vi "Obtain Request Events.vi"(8 "error in":errorcluster, 10 "Create New? (F)":bool, 11 "Module ID":i32=-1) -> (0 "error out":errorcluster, 2 "RaspberryPiPico Request Events":T1)   [LabVIEW 2024, in "RaspberryPiPico.lvlib"]
doc: "This VI Obtains/Creates the Requests events that will be used for other modules to communicate with the module that owns this VI. These Requests events will be accessed only via Public API methods for this module.\n\n<b>NOTE</b>: The contents of this VI are automatically generated and modified by the <b>Tools > DQMH Consortium > DQMH</b> utilities. Consider using those utilities instead of making your own modifications to this VI.\n_____\nBased on DQMH Dev Tools: Project Template 7.1.0.1503."
uses:
  RaspberryPiPico.lvlib
  Request Events--cluster.ctl
  Stop Argument--cluster.ctl
  Show Panel Argument--cluster.ctl
  Hide Panel Argument--cluster.ctl
  Show Diagram Argument--cluster.ctl
  Get Module Execution Status Argument--cluster.ctl
  Initialize Instrument Argument--cluster.ctl
  Initialize Instrument (Reply Payload)--cluster.ctl
  <instrlib>/HandsOnPi2040/cti-drivers-lv-visa-main/CTI-Visa/Identity.ctl
  Local Instance Request Events--cluster.ctl
  Start Continuous Acquisition Argument--cluster.ctl
  <instrlib>/HandsOnPi2040/cti-drivers-lv-visa-main/CTI-Visa/CTI-Visa.lvlib
  Local Instance Events SEQ/Local Instance Events SEQ.lvlib
panel:
  # "NOTE: The contents of this VI are automatically generated and modified by the Tools > DQMH Consortium > DQMH utilities. Consider using those utilities instead of making your own modifications to this VI."
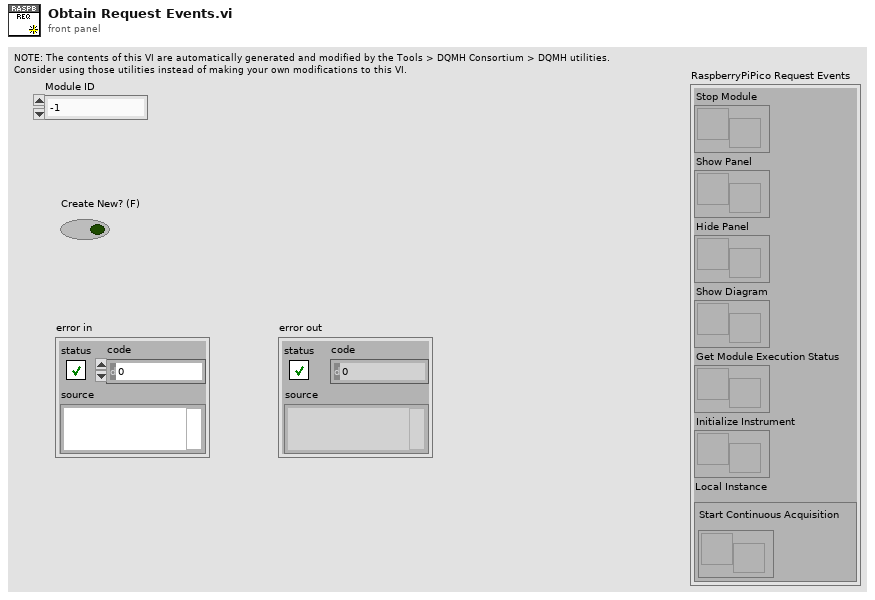
[diagram p1: front panel]
types:
  T1 = typedef "RaspberryPiPico.lvlib/Request Events--cluster.ctl" = cluster{"Stop Module":refnum<user-event>, "Show Panel":refnum<user-event>, "Hide Panel":refnum<user-event>, "Show Diagram":refnum<user-event>, "Get Module Execution Status":refnum<user-event>, "Initialize Instrument":refnum<user-event>, "Local Instance":T2}
  T2 = typedef "RaspberryPiPico.lvlib/Local Instance Request Events--cluster.ctl" = cluster{"Start Continuous Acquisition":refnum<user-event>}
  T3 = typedef "RaspberryPiPico.lvlib/Initialize Instrument Argument--cluster.ctl" = cluster{"Module ID":i32, "VISA resource name":refnum<visa-resource-name>, "Wait Notifier":refnum<notifier>, "wait for reply":bool}
  T4 = typedef "RaspberryPiPico.lvlib/Get Module Execution Status Argument--cluster.ctl" = cluster{"Module ID":i32, "Running?":bool}
  T5 = typedef "RaspberryPiPico.lvlib/Show Diagram Argument--cluster.ctl" = cluster{"Module ID":i32, "Debug?":bool}
  T6 = typedef "RaspberryPiPico.lvlib/Show Panel Argument--cluster.ctl" = cluster{"Module ID":i32, "Show Panel?":bool}
  T7 = typedef "RaspberryPiPico.lvlib/Hide Panel Argument--cluster.ctl" = cluster{"Module ID":i32, "Hide Panel?":bool}
  T8 = typedef "RaspberryPiPico.lvlib/Stop Argument--cluster.ctl" = cluster{"Module ID":i32, "Origin":string, "Exit via Stop Module Req?":bool, "Wait for Module to stop?":bool}
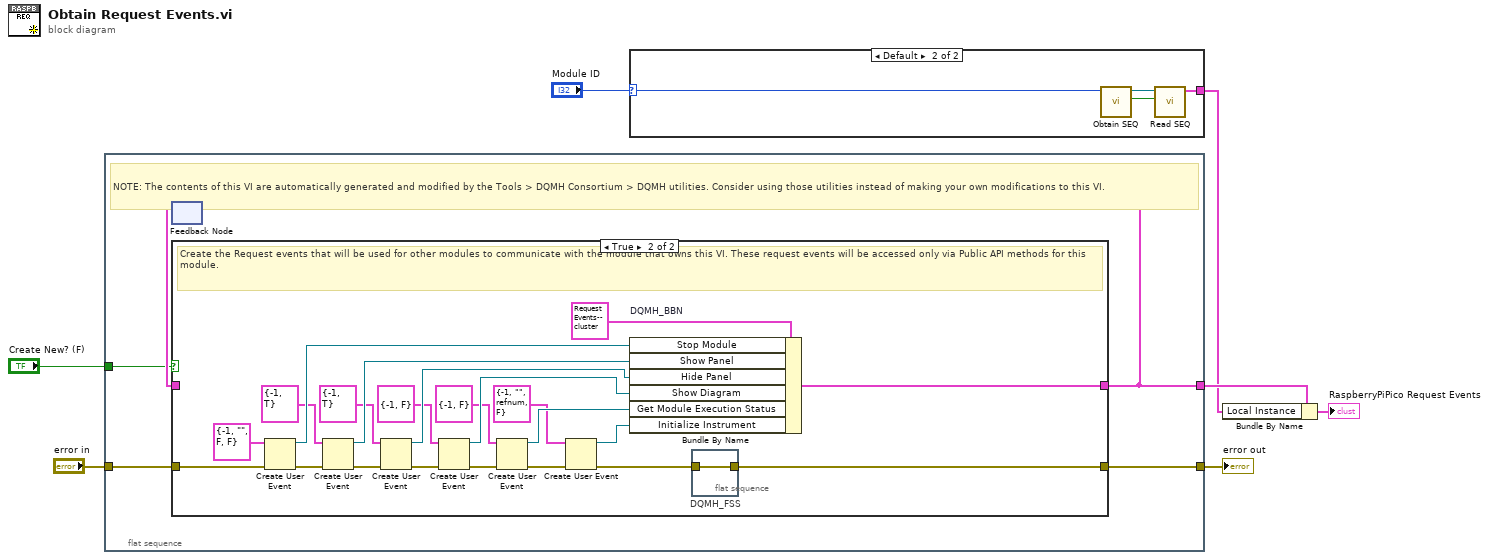
[diagram p0: block diagram]
diagram:
  n1 = flat-sequence {
    tunnel: [w12] -> w7
    tunnel: "error in" -> [w11]
    tunnel: [w9] -> w3
    tunnel: "Create New? (F)" -> [w8]
    frame #0 {
      # "NOTE: The contents of this VI are automatically generated and modified by the Tools > DQMH Consortium > DQMH utilities. Consider using those utilities instead of making your own modifications to this VI."
      n2 = feedback #1() -> (w10:T1)  [unwired: 1 in]
      n3 = case shown="True" w8 {
        tunnel: [w13 w24] -> w12
        tunnel: w11 -> [w13 w36]
        tunnel: [w14 w33] -> w9
        tunnel: w10 -> [w14 _]
        frame False {
        }
        frame True {
          # "Create the Request events that will be used for other modules to communicate with the module that owns this VI. These request events will be accessed only via Public API methods for this module."
          n4 = Create User Event(user event datatype=T8 {"Module ID"=-1, "Origin"="", "Exit via Stop Module Req?"=FALSE, "Wait for Module to stop?"=FALSE} ("Stop Argument"), error in=w36) -> (user event=w34:refnum<user-event>, error out=w31:errorcluster)
          n5 = Create User Event(user event datatype=T6 {"Module ID"=-1, "Show Panel?"=TRUE} ("Show Panel Argument"), error in=w31) -> (user event=w30:refnum<user-event>, error out=w28:errorcluster)
          n6 = Create User Event(user event datatype=T7 {"Module ID"=-1, "Hide Panel?"=TRUE} ("Hide Panel"), error in=w28) -> (user event=w27:refnum<user-event>, error out=w26:errorcluster)
          n7 = Create User Event(user event datatype=T5 {"Module ID"=-1, "Debug?"=FALSE} ("Show Diagram Argument"), error in=w26) -> (user event=w22:refnum<user-event>, error out=w23:errorcluster)
          n8 = Create User Event(user event datatype=T4 {"Module ID"=-1, "Running?"=FALSE} ("Get Module Execution Status Argument"), error in=w23) -> (user event=w19:refnum<user-event>, error out=w20:errorcluster)
          n9 = Create User Event(user event datatype=T3 {"Module ID"=-1, "VISA resource name"="", "Wait Notifier"=refnum, "wait for reply"=FALSE} ("Initialize Instrument Argument"), error in=w20) -> (user event=w16:refnum<user-event>, error out=w17:errorcluster)
          n10 = Bundle By Name "DQMH_BBN"(cluster=T1 {"Stop Module"=refnum, "Show Panel"=refnum, "Hide Panel"=refnum, "Show Diagram"=refnum, "Get Module Execution Status"=refnum, "Initialize Instrument"=refnum, "Local Instance"={"Start Continuous Acquisition"=refnum}} ("output cluster"), "Stop Module"=w34, "Show Panel"=w30, "Hide Panel"=w27, "Show Diagram"=w22, "Get Module Execution Status"=w19, "Initialize Instrument"=w16) -> (w33:T1)
          n11 = flat-sequence "DQMH_FSS" {
            tunnel: w17 -> [w37]
            tunnel: [w37] -> w24
            frame #0 {
            }
          }
        }
      }
      n12 = feedback-in #1(w9) -> ()
    }
  }
  n13 = case shown="Default" "Module ID" {
    selector: "Module ID" -> [_ w39]
    tunnel: [_ w38] -> w2
    frame -1 {
    }
    frame Default {
      n14 = call "Obtain SEQ.vi"("Module ID"=w39) -> ("Created New?"=w40:bool, "Local Instance Event SEQ"=w41:refnum<queue>)  [unwired: 8 in, 1 out]
      n15 = call "Read SEQ.vi"("Created New?"=w40, "Local Instance Event SEQ"=w41) -> ("Local Instance Request Events"=w38:T2)  [unwired: 8 in, 1 out]
    }
  }
  n16 = Bundle By Name(cluster=w3, "Local Instance"=w2) -> (→"RaspberryPiPico Request Events":T1)
  "error out" <- w7
